vi "Find (Create) Object.vi"(7 "Object Path":string, 8 "error in (no error)":errorcluster, 10 "Starting Offset":i32, 11 "JSON":string="{}") -> (0 "error out":errorcluster, 2 "Object offset":i32, 3 "<JSON>":string caption="<JSON> (possibly with empty object inserted)")   [LabVIEW 2020, in "JSONtext.lvlib"]
doc: "Ensures that a JSON Object exists at Path, and returns the offset to that object. If the object does not exist but it's parent object does, then an empty object is inserted. An error is output if a non-object exists at the specified path."
uses:
  <vilib>/JDP Science/JSONtext/JSONtext.lvlib
  <vilib>/JDP Science/JSONtext/Parsing/Replace at Offset.vi
  <vilib>/JDP Science/JSONtext/support/Make empty strings null.vi
  <vilib>/JDP Science/JSONtext/Parsing/Advance past Line Ending.vi
  <vilib>/JDP Science/JSONtext/Parsing/Parse Path Object Items.vi
  <vilib>/JDP Science/JSONtext/Parsing/Advance past replacable whitespace.vi
  <vilib>/JDP Science/JSONtext/Parsing/Match Pattern.vi
  <vilib>/JDP Science/JSONtext/support/Quote and Escape JSON string.vi
  <vilib>/JDP Science/JSONtext/Parsing/Advance past String.vi
  <vilib>/JDP Science/JSONtext/Parsing/Advance past whitespace and comma.vi
  <vilib>/JDP Science/JDP Science Common Utilities/Trim Whitespace__JDP.vi
  <vilib>/JDP Science/JSONtext/support/quote and escape json string 2.vi
  <vilib>/JDP Science/JSONtext/Parsing/Parsing Error.vi
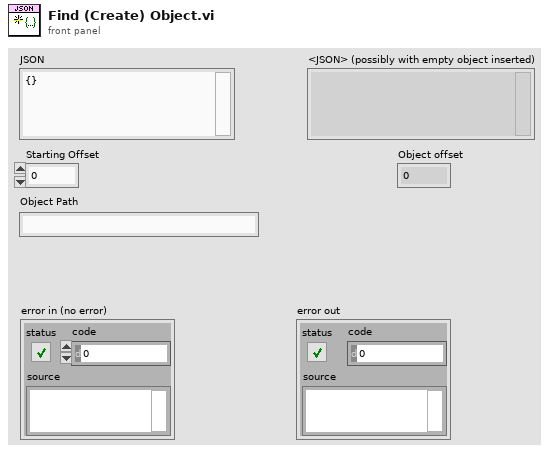
[diagram p1: front panel]
types:
  T1 = typedef "JSONtext.lvlib/Found Items.ctl" = cluster{"Item offset":i32, "Offset past Item":i32, "Name offset":i32, "Offset past Name":i32, "Found":bool, "Item Type":T2, "Item Index":i32, "Start Offset":i32, "Comma Needed For Insert":T3}
  T2 = typedef "JSONtext.lvlib/Parsing State.ctl" = enum16{"Parser Error", "Object", "Array", "String", "Number/Other", "Leading Whitespace", "Object end", "Array end", "Value end"}
  T3 = typedef "JSONtext.lvlib/Comma Needed for Insert.ctl" = enum8{"False", "True", "Following"}
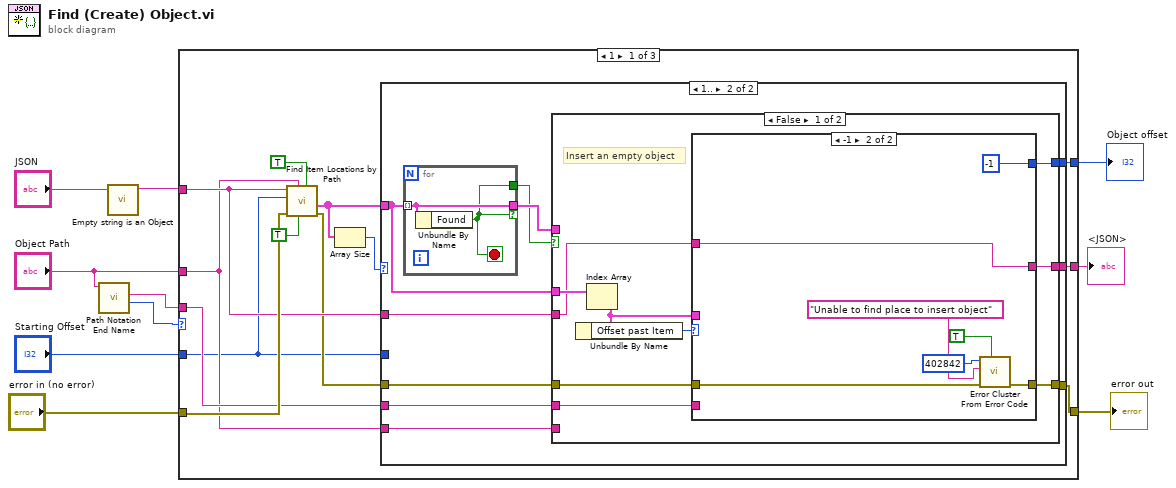
[diagram p0: block diagram]
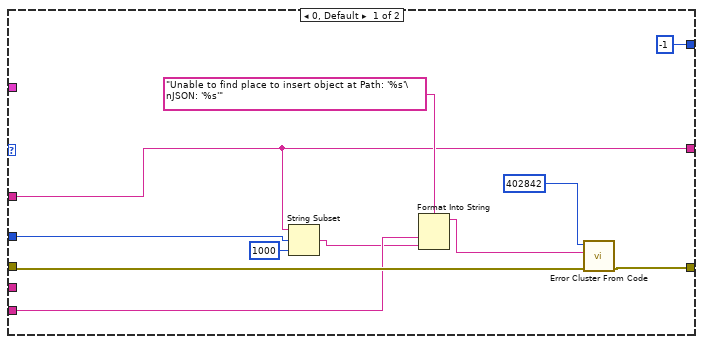
[diagram p2: hidden frame]
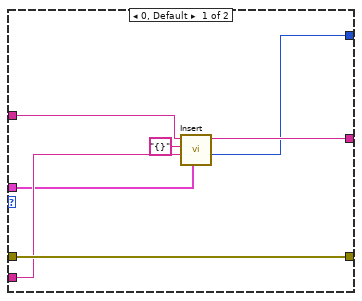
[diagram p3: hidden frame]
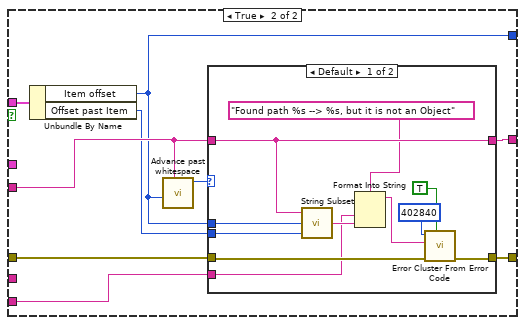
[diagram p4: hidden frame]
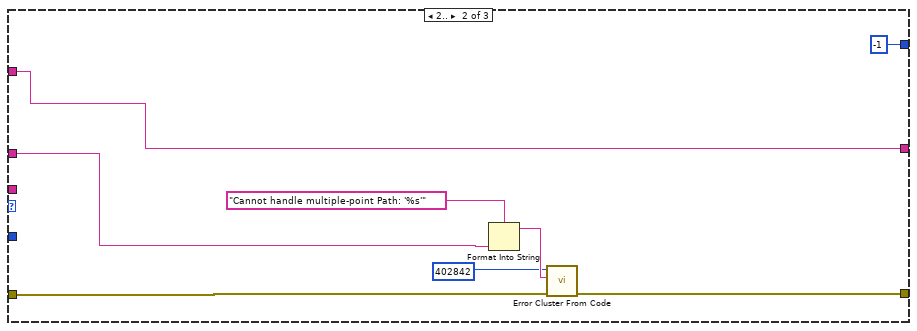
[diagram p6: hidden frame]
diagram:
  n1 = call <vilib>:"Path Notation End Name.vi"("Item Path"="Object Path") -> ("Number of Paths"=w1:i32, "<JSON>End Name"=w6:string)  [unwired: 8 in, 1 out]
  n2 = call <vilib>:"Empty string is an Object.vi"("JSON Input"="JSON") -> ("<JSON>Object"=w2:string)  [unwired: 10 in]
  n3 = case shown="1" w1 {
    tunnel: "Object Path" -> [w14 w98 _]
    tunnel: "Starting Offset" -> [w11 _ w101]
    tunnel: "error in (no error)" -> [w23 w94 w100]
    tunnel: [w17 w93 w100] -> w8
    tunnel: w2 -> [w22 w96 w102]
    tunnel: [w20 -1 ("Item offset") w101] -> w7
    tunnel: w6 -> [w16 _ _]
    tunnel: [w15 w96 w102] -> w4
    frame 1 {
      n4 = call <vilib>:"Find Item Locations by Path.vi"("Insertion point if not found"=TRUE, "Only return first found"=TRUE, "Path"=w14, "error in (no error)"=w23, "Offset"=w11, "JSON"=w22) -> ("error out"=w18:errorcluster, "Items"=w13:T1[])  [unwired: 4 in]
      n5 = Array Size(array=w13) -> (size(s)=w12:i32)
      n6 = case shown="1.." w12 {
        tunnel: w22 -> [w28 w44]
        tunnel: [-1 ("Item offset") w42] -> w20
        tunnel: w18 -> [w33 w40]
        tunnel: [w31 w39] -> w17
        tunnel: w16 -> [_ w38]
        tunnel: [w28 w37] -> w15
        tunnel: w14 -> [w29 w36]
        tunnel: w13 -> [_ w35]
        tunnel: w11 -> [w24 _]
        frame 0, Default {
          n7 = String Subset(string=w28, offset (0)=w24, length (rest)=1000 ("length (rest)")) -> (substring=w27:string)
          n8 = Format Into String(format string="Unable to find place to insert object at Path: '%s'\nJSON: '%s'", w29, w27) -> (resulting string=w25:string)  [unwired: 2 in, 1 out]
          n9 = call <vilib>:"Error Cluster From Code.vi"("error in (no error)"=w33, "error message (\"\")"=w25, "error code (402840+)"=402842 ("error code (0)")) -> ("error out"=w31:errorcluster)  [unwired: 6 in]
        }
        frame 1.. {
          n10 = for {
            tunnel: w35 -> [w91] mode=indexing
            tunnel: [w91] -> w43 if=w90
            tunnel: [w90] -> w41
            stop <- w90 stop-if-true
            n11 = Unbundle By Name(w91) -> ("Found"=w90:bool)
          }
          n12 = case shown="False" w41 {
            tunnel: w44 -> [w49 w71]
            tunnel: w43 -> [_ w76]
            tunnel: [w45 w70] -> w42
            tunnel: w40 -> [w50 w73]
            tunnel: [w51 w74] -> w39
            tunnel: w35 -> [w53 _]
            tunnel: w38 -> [w48 _]
            tunnel: [w46 w72] -> w37
            tunnel: w36 -> [_ w68]
            frame False {
              # "Insert an empty object"
              n13 = Index Array(array=w53) -> (element=w47:T1)  [unwired: 1 in]
              n14 = Unbundle By Name(w47) -> ("Offset past Item"=w52:i32)
              n15 = case shown="-1" w52 {
                tunnel: [w60 w67] -> w51
                tunnel: w50 -> [w60 w66]
                tunnel: w49 -> [w59 w62]
                tunnel: w48 -> [w58 _]
                tunnel: w47 -> [w56 _]
                tunnel: [w55 w62] -> w46
                tunnel: [w54 -1 ("Item offset")] -> w45
                frame 0, Default {
                  n16 = call <vilib>:"Insert.vi"("Item"=w56, "<JSON>name"=w58, "JSON to Insert"="{}", "JSON in"=w59) -> ("Inserted Item Offset"=w54:i32, "string"=w55:string)  [unwired: 5 in, 1 out]
                }
                frame -1 {
                  n17 = call <vilib>:"Error Cluster From Error Code.vi"("show call chain? (False)"=TRUE, "error in (no error)"=w66, "error message (\"\")"="Unable to find place to insert object", "error code (0)"=402842) -> ("error out"=w67:errorcluster)  [unwired: 5 in]
                }
              }
            }
            frame True {
              n18 = Unbundle By Name(w76) -> ("Item offset"=w70:i32, "Offset past Item"=w69:i32)
              n19 = call <vilib>:"Advance past whitespace.vi"("JSON"=w71, "Offset"=w70) -> ("Parser State"=w75:T2)  [unwired: 7 in, 2 out]
              n20 = case shown="Default" w75 {
                tunnel: [w87 w89] -> w74
                tunnel: w73 -> [w86 w89]
                tunnel: [w83 w88] -> w72
                tunnel: w71 -> [w83 w88]
                tunnel: w70 -> [w82 _]
                tunnel: w69 -> [w81 _]
                tunnel: w68 -> [w77 _]
                frame Default {
                  n21 = call <vilib>:"String Subset.vi"("Offset past End"=w81, "Start offset"=w82, "JSON"=w83) -> ("substring"=w79:string)  [unwired: 2 in]
                  n22 = Format Into String(format string="Found path %s --> %s, but it is not an Object" ("error message (\"\")"), w77, w79) -> (resulting string=w78:string)  [unwired: 2 in, 1 out]
                  n23 = call <vilib>:"Error Cluster From Error Code.vi"("show call chain? (False)"=TRUE, "error in (no error)"=w86, "error message (\"\")"=w78, "error code (0)"=402840) -> ("error out"=w87:errorcluster)  [unwired: 5 in]
                }
                frame "Object" {
                }
              }
            }
          }
        }
      }
    }
    frame 2.. {
      n24 = Format Into String(format string="Cannot handle multiple-point Path: '%s'", w98) -> (resulting string=w95:string)  [unwired: 2 in, 1 out]
      n25 = call <vilib>:"Error Cluster From Code.vi"("error in (no error)"=w94, "error message (\"\")"=w95, "error code (402840+)"=402842 ("error code (0)")) -> ("error out"=w93:errorcluster)  [unwired: 6 in]
    }
    frame ..0 {
    }
  }
  "error out" <- w8
  "Object offset" <- w7
  "<JSON>" <- w4
